vi "Write StopVelocity.vi"(8 "error in (no error)":errorcluster, 10 "StopVelocity":dbl, 11 "Configure StopVelocity Msg in":refnum<class "Configure StopVelocity Msg.lvclass">) -> (0 "error out":errorcluster, 3 "Configure StopVelocity Msg out":refnum<class "Configure StopVelocity Msg.lvclass">)   [LabVIEW 2015, in "CS++Motor.lvlib" / "Configure StopVelocity Msg.lvclass"]
uses:
  Configure StopVelocity Msg.lvclass
  Configure StopVelocity Msg.lvclass/Configure StopVelocity Msg.ctl
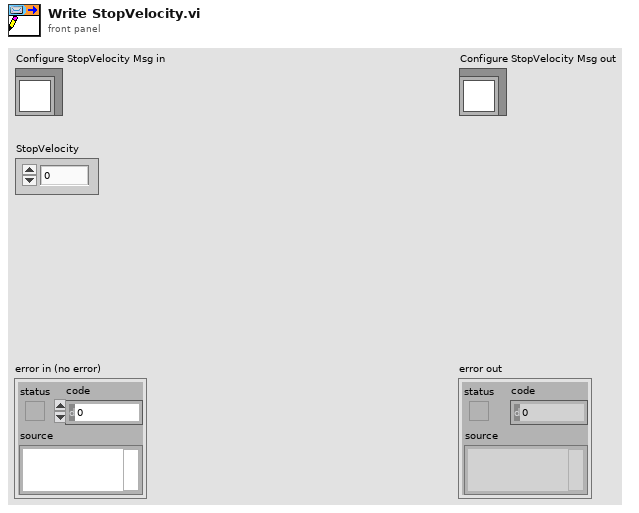
[diagram p1: front panel]
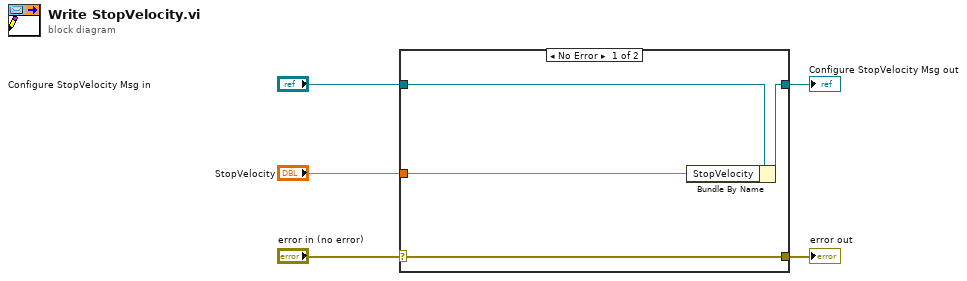
[diagram p0: block diagram]
diagram:
  n1 = case shown="No Error" "error in (no error)" {
    selector: "error in (no error)" -> [w9 w10]
    tunnel: [w9 w10] -> w4
    tunnel: [w7 w11] -> w2
    tunnel: "Configure StopVelocity Msg in" -> [w8 w11]
    tunnel: "StopVelocity" -> [w6 _]
    frame No Error {
      n2 = Bundle By Name(cluster=w8, "StopVelocity"=w6) -> (w7:refnum<class "Configure StopVelocity Msg.lvclass">)
    }
    frame Error {
    }
  }
  "error out" <- w4
  "Configure StopVelocity Msg out" <- w2
